vi "Set-Query SRER.vi"(8 "error   in (no error)":errorcluster caption="error  in (no error)" {"code" format="%.0x"}, 9 "Enable SRER":T1, 10 "Enable Mask (T)":bool=TRUE, 11 "VISA session":refnum<visa-resource-name>) -> (0 "error out":errorcluster {"code" format="%.0x"}, 1 "Read SRER":T2, 3 "dup VISA session":refnum<visa-resource-name>)   [LabVIEW 2011]
doc: "Sets or queries the bits in the instrument's IEEE-488.2 Service Request Enable Register.\n\nNote: Reading the SRER reads the current mask status. To read the actual value of the Status Byte Register (STB), call the Check SBR.vi."
uses:
  Low Level/Status Byte Indicator.ctl
  Low Level/Service Request Enable Control.ctl
panel:
  # "service request enable register (SRER)"
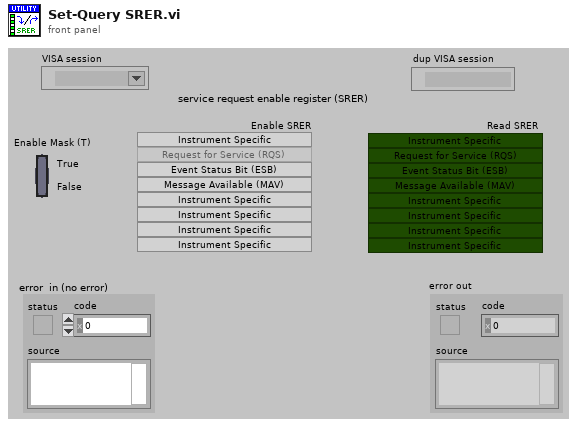
[diagram p1: front panel]
types:
  T1 = typedef "Service Request Enable Control.ctl" = cluster{" Instrument Specific (1)":bool, " Instrument Specific (2)":bool, " Instrument Specific (4)":bool, " Instrument Specific (8)":bool, "Message Available (16)":bool, "Event Status Bit (32)":bool, "Request for Service (64)":bool, " Instrument Specific (128)":bool}
  T2 = typedef "Status Byte Indicator.ctl" = cluster{"Instrument Specific (1)":bool, "Instrument Specific (2)":bool, "Instrument Specific (4)":bool, "Instrument Specific (8)":bool, "Message Available (16)":bool, "Event Status Bit (32)":bool, "Request for Service (32)":bool, "Instrument Specific (128)":bool}
  T3 = cluster{" Instrument Specific (1)":bool, " Instrument Specific (2)":bool, " Instrument Specific (4)":bool, " Instrument Specific (8)":bool, "Message Available (16)":bool, "Event Status Bit (32)":bool, bool, " Instrument Specific (128)":bool}
  T4 = cluster{"[0]":bool, "[1]":bool, "[2]":bool, "[3]":bool, "[4]":bool, "[5]":bool, "[6]":bool, "[7]":bool}
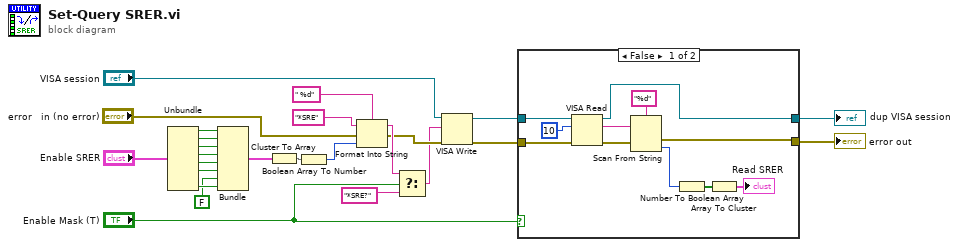
[diagram p0: block diagram]
diagram:
  n1 = Unbundle("Enable SRER") -> ("Instrument Specific (1)"=w24:bool, "Instrument Specific (2)"=w23:bool, "Instrument Specific (4)"=w22:bool, "Instrument Specific (8)"=w21:bool, "Message Available (16)"=w20:bool, "Event Status Bit (32)"=w19:bool, "Instrument Specific (128)"=w18:bool)  [unwired: 1 out]
  n2 = Bundle("Instrument Specific (1)"=w24, "Instrument Specific (2)"=w23, "Instrument Specific (4)"=w22, "Instrument Specific (8)"=w21, "Message Available (16)"=w20, "Event Status Bit (32)"=w19, FALSE, "Instrument Specific (128)"=w18) -> (w15:T3)  [unwired: 1 in]
  n3 = Cluster To Array(cluster=w15) -> (array=w25:bool[])
  n4 = Boolean Array To Number(Boolean array=w25) -> (number=w5:u32)
  n5 = Format Into String(format string=" %d", initial string="*SRE", error in="error   in (no error)", w5) -> (resulting string=w3:string, error out=w2:errorcluster)
  n6 = Select(t=w3, s="Enable Mask (T)", f="*SRE?") -> (s? t:f=w1:string)
  n7 = VISA Write(VISA resource name="VISA session", write buffer=w1, error in (no error)=w2) -> (VISA resource name out=w12:refnum<visa-resource-name>, error out=w13:errorcluster)  [unwired: 1 out]
  n8 = case shown="False" "Enable Mask (T)" {
    tunnel: w13 -> [w32 w38]
    tunnel: w12 -> [w33 w37]
    tunnel: [w27 w38] -> w11
    tunnel: [w26 w37] -> w7
    frame False {
      n9 = VISA Read(VISA resource name=w33, byte count=10, error in (no error)=w32) -> (VISA resource name out=w26:refnum<visa-resource-name>, read buffer=w29:string, error out=w28:errorcluster)  [unwired: 1 out]
      n10 = Scan From String(format string="%d", input string=w29, error in=w28) -> (error out=w27:errorcluster, output 1=w31:i32)  [unwired: 2 in, 2 out]
      n11 = Number To Boolean Array(number=w31) -> (Boolean array=w36:bool[])
      n12 = Array To Cluster(array=w36) -> (cluster=→"Read SRER":T4)
    }
    frame True {
    }
  }
  "error out" <- w11
  "dup VISA session" <- w7
